vi "Load Configuration.vi"(0 "INI Station Configuration in":T1, 5 "INI file path in":path, 11 "error in":errorcluster) -> (4 "INI Station Configuration out":T1, 15 "error out":errorcluster)   [LabVIEW 2016, in "TLB` Template.lvlib" / "{TMPL} Station Configuration.lvclass"]
uses:
  {TMPL} Station Configuration.lvclass
  {TMPL} Station Configuration.lvclass/{TMPL} Station Configuration.ctl
  <vilib>/Utility/config.llb/Read Key (String).vi
  <vilib>/Utility/config.llb/NI_LVConfig.lvlib
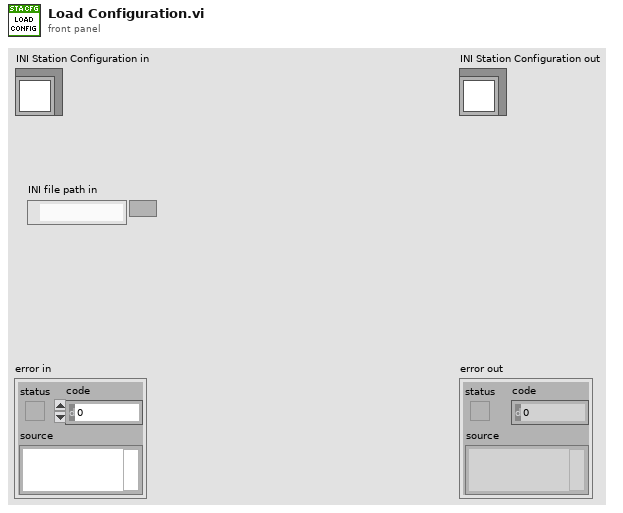
[diagram p1: front panel]
types:
  T1 = refnum<class "{TMPL} Station Configuration.lvclass">
  T2 = typedef "NI_LVConfig.lvlib/Config Data RefNum.ctl" = refnum<k1>
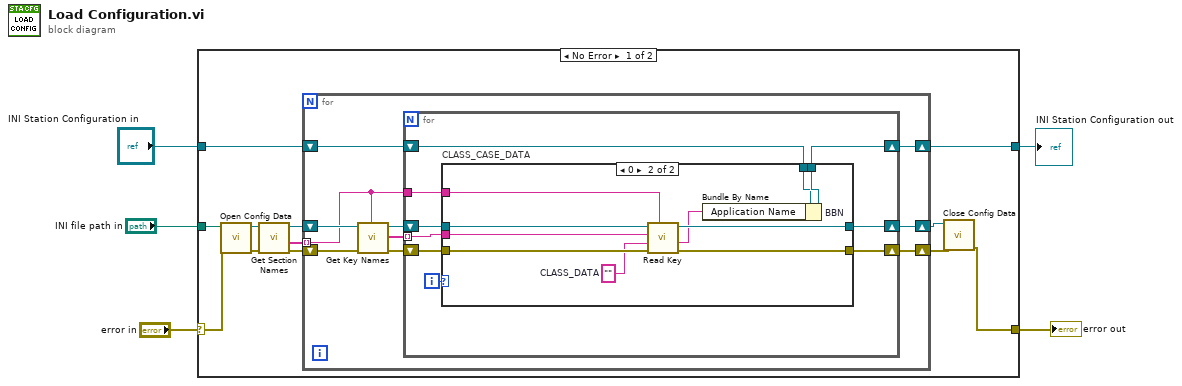
[diagram p0: block diagram]
diagram:
  n1 = case shown="No Error" "error in" {
    selector: "error in" -> [w13 w49]
    tunnel: [w16 w48] -> w2
    tunnel: [w8 w49] -> w1
    tunnel: "INI Station Configuration in" -> [w15 w48]
    tunnel: "INI file path in" -> [w14 _]
    frame No Error {
      n2 = call <vilib>:"Open Config Data.vi"("error in (no error)"=w13, "configuration file path"=w14) -> ("error out"=w12:errorcluster, "refnum"=w11:T2)  [unwired: 7 in, 1 out]
      n3 = call <vilib>:"Get Section Names.vi"("refnum"=w11) -> ("section names"=w6:string[], "refnum out"=w7:T2)  [unwired: 8 in, 1 out]
      n4 = for {
        shift-right: [w25] -> w16
        shift-left: w15 -> [w24]
        shift-right: [w20] -> w9
        shift-left: w12 -> [w23]
        shift-right: [w21] -> w10
        shift-left: w7 -> [w22]
        tunnel: w6 -> [w18] mode=indexing
        n5 = call <vilib>:"Get Key Names.vi"("section"=w18, "refnum"=w22) -> ("key names"=w17:string[], "refnum out"=w19:T2)  [unwired: 6 in, 2 out]
        n6 = for {
          shift-right: [w33] -> w25
          shift-left: w24 -> [w28]
          shift-right: [w30] -> w20
          shift-left: w23 -> [w32]
          shift-right: [w29] -> w21
          shift-left: w19 -> [w31]
          tunnel: w18 -> [w27]
          tunnel: w17 -> [w26] mode=indexing
          i -> [w34]
          n7 = case "CLASS_CASE_DATA" shown="0" w34 {
            tunnel: [w35 w41] -> w33
            tunnel: w32 -> [w36 w46]
            tunnel: w31 -> [w37 w47]
            tunnel: [w36 w44] -> w30
            tunnel: [w37 w43] -> w29
            tunnel: w28 -> [w35 w38]
            tunnel: w27 -> [_ w40]
            tunnel: w26 -> [_ w39]
            frame Default {
            }
            frame 0 {
              w45 = ""  # CLASS_DATA
              n8 = call-poly <vilib>:"Read Key.vi"("section"=w40, "error in (no error)"=w46, "default value"=w45, "key"=w39, "refnum"=w47) -> ("error out"=w44:errorcluster, "value"=w42:string, "refnum out"=w43:T2)  [unwired: 3 in, 1 out]
              n9 = Bundle By Name "BBN"(cluster=w38, "Application Name"=w42) -> (w41:T1)
            }
          }
        }
      }
      n10 = call <vilib>:"Close Config Data.vi"("error in (no error)"=w9, "refnum"=w10) -> ("error out"=w8:errorcluster)  [unwired: 8 in, 1 out]
    }
    frame Error {
    }
  }
  "error out" <- w1
  "INI Station Configuration out" <- w2
